vi "URAPIFirmwareTest.vi"(3 "error in":errorcluster, 4 "Task":enum16{"Get Version", "Replace"}(ring), 5 "Bot Settings":T1) -> (0 "error out":errorcluster, 1 "Version":dbl, 2 "Bot Settings":T1)   [LabVIEW 2014]
uses:
  <userlib>/botspeakLib/VIs/Direct/BotSpeak_Control.ctl
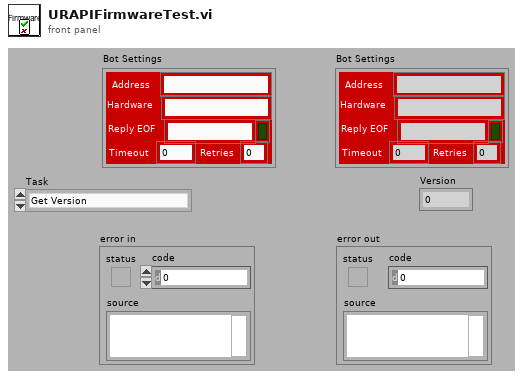
[diagram p1: front panel]
types:
  T1 = typedef "BotSpeak_Control.ctl" = cluster{"Address":string, "Reply EOF":string, "Hardware":string, "Retries":i8, "Timeout":i32, "Open?":bool}
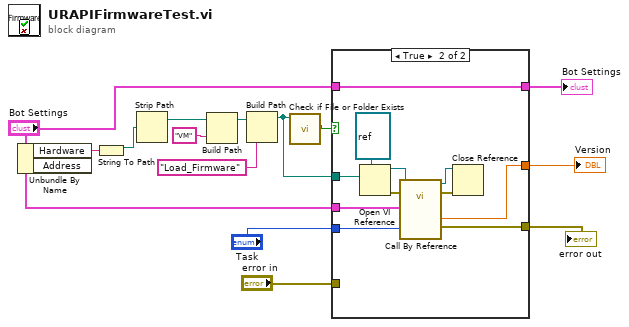
[diagram p0: block diagram]
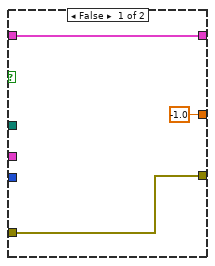
[diagram p2: hidden frame]
diagram:
  n1 = Unbundle By Name("Bot Settings") -> ("Hardware"=w9:string)  [unwired: 1 out]
  n2 = String To Path(string=w9) -> (path=w7:path)
  n3 = Strip Path(path=w7) -> (stripped path=w8:path)  [unwired: 1 out]
  n4 = Build Path(base path=w8, name or relative path="VM") -> (appended path=w13:path)
  n5 = Build Path(base path=w13, name or relative path="Load_Firmware") -> (appended path=w11:path)
  n6 = call <vilib>:"Check if File or Folder Exists.vi"("path"=w11) -> ("file or folder exists?"=w10:bool)  [unwired: 8 in, 2 out]
  n7 = case shown="True" w10 {
    tunnel: [w17 w22] -> w12
    tunnel: w11 -> [_ w23]
    tunnel: [w16 w21] -> w6
    tunnel: "Bot Settings" -> [w16 w21]
    tunnel: "error in" -> [w17 _]
    tunnel: "Bot Settings" -> [_ w20]
    tunnel: "Task" -> [_ w19]
    tunnel: [-1.0 ("Version") w18] -> w1
    frame False {
    }
    frame True {
      n8 = Open VI Reference(type specifier VI Refnum (for type only)=refnum<vi> refnum, vi path=w23) -> (vi reference=w28:refnum<vi>, error out=w27:errorcluster)  [unwired: 4 in]
      n9 = call-by-ref "?"(reference=w28, error in=w27, "Task"=w19, "Bot Settings"=w20) -> (reference out=w25:refnum<vi>, error out=w26:errorcluster, 0:"error out"=w22:errorcluster, "Version"=w18:dbl)  [unwired: 1 in, 1 out]
      n10 = Close Reference(reference=w25, error in (no error)=w26) -> ()  [unwired: 1 out]
    }
  }
  "error out" <- w12
  "Bot Settings" <- w6
  "Version" <- w1
